vi "libssh2_knownhost_checkp.vi"(5 "port":i32, 7 "host":string, 8 "error in (no error)":errorcluster, 9 "typemask":i32, 10 "key":u8[](array[numeric]), 11 "Hosts":T2) -> (0 "error out":errorcluster, 2 "Host":T1, 3 "return value":i32)   [LabVIEW 2013, in "libssh2.lvlib"]
uses:
  libssh2.lvlib
  Hosts Refnum.ctl
  Host Refnum.ctl
  libssh2.dll
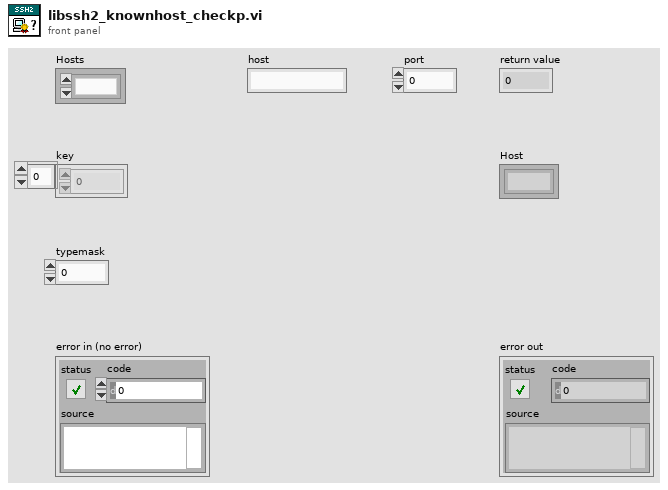
[diagram p1: front panel]
types:
  T1 = typedef "libssh2.lvlib/Host Refnum.ctl" = refnum<k1>
  T2 = typedef "libssh2.lvlib/Hosts Refnum.ctl" = refnum<k1>
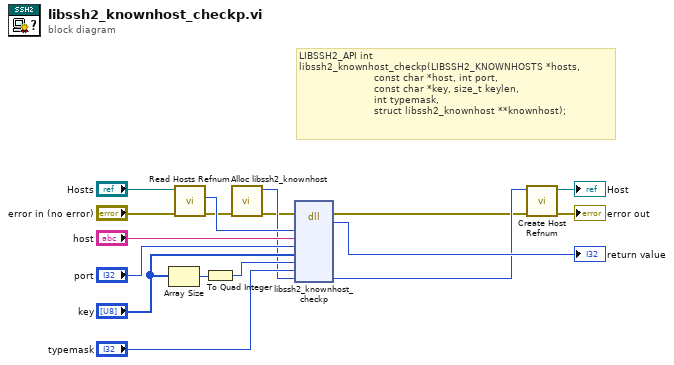
[diagram p0: block diagram]
diagram:
  # "LIBSSH2_API int\nlibssh2_knownhost_checkp(LIBSSH2_KNOWNHOSTS *hosts,\n                         const char *host, int port,\n                         const char *key, size_t keylen,\n                         int typemask,\n                         struct libssh2_knownhost **knownhost);"
  n1 = Array Size(array="key") -> (size(s)=w14:i32)
  n2 = call "Read Hosts Refnum.vi"("error in (no error)"="error in (no error)", "Hosts"="Hosts") -> ("error out"=w7:errorcluster, "LIBSSH2_KNOWNHOSTS*"=w8:u64)  [unwired: 8 in]
  n3 = To Quad Integer(1:w14) -> (0:w13:i64)
  n4 = call "Alloc libssh2_knownhost.vi"("error in (no error)"=w7) -> ("error out"=w5:errorcluster, "libssh2_knownhost*"=w6:u64)  [unwired: 9 in]
  n5 = dll-call lib="C:/Users/pasca/source/repos/libssh2-labview/libssh2**.*" fn="libssh2_knownhost_checkp"(error in=w5, "hosts"=w8, "host"="host", "port"="port", "key"="key", "keylen"=w13, "typemask"="typemask", "knownhost"=w6) -> (error out=w1:errorcluster, "return value"=→"return value":i32, "knownhost"=w3:u64)  [unwired: 8 in, 1 out]
  n6 = call "Create Host Refnum.vi"("error in (no error)"=w1, "libssh2_knownhost*"=w3) -> ("error out"=→"error out":errorcluster, "Host"=→"Host":T1)  [unwired: 8 in]
